vi "Main.vi"   [LabVIEW 2020, in "ClashRoyale.lvclass"]
uses:
  ClashRoyale.lvclass
  support/Popup Loading Toolkit.lvlibp/Handler/Popup Loading Handler.lvclass
types:
  T1 = typedef "InitParameters.ctl" = cluster{"PlayerTag":string}
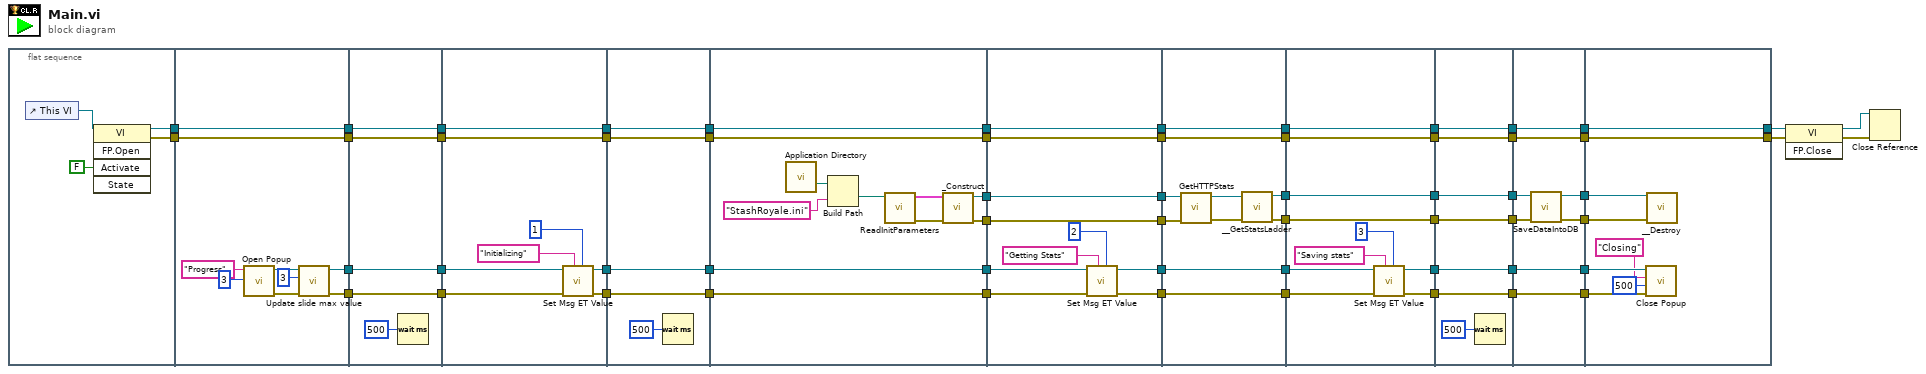
[diagram p0: block diagram]
diagram:
  n1 = flat-sequence {
    tunnel: [w61] -> w16
    tunnel: [w60] -> w5
    tunnel: [w68] -> w38
    tunnel: [w67] -> w36
    tunnel: [w64] -> w17
    tunnel: w16 -> [w64]
    tunnel: [w63] -> w6
    tunnel: w5 -> [w63]
    tunnel: w38 -> [w76]
    tunnel: [w76] -> w37
    tunnel: w36 -> [w75]
    tunnel: [w75] -> w35
    tunnel: [w73] -> w18
    tunnel: w17 -> [w73]
    tunnel: [w72] -> w7
    tunnel: w6 -> [w72]
    tunnel: w37 -> [w84]
    tunnel: w35 -> [w83]
    tunnel: [w80] -> w42
    tunnel: [w79] -> w40
    tunnel: [w78] -> w19
    tunnel: w18 -> [w78]
    tunnel: [w77] -> w8
    tunnel: w7 -> [w77]
    tunnel: w42 -> [w89]
    tunnel: [w89] -> w41
    tunnel: w40 -> [w88]
    tunnel: [w88] -> w39
    tunnel: [w86] -> w20
    tunnel: w19 -> [w86]
    tunnel: [w85] -> w9
    tunnel: w8 -> [w85]
    tunnel: w41 -> [w93]
    tunnel: w39 -> [w92]
    tunnel: [w95] -> w58
    tunnel: [w94] -> w57
    tunnel: [w93] -> w56
    tunnel: [w92] -> w55
    tunnel: [w91] -> w21
    tunnel: w20 -> [w91]
    tunnel: [w90] -> w10
    tunnel: w9 -> [w90]
    tunnel: w58 -> [w110]
    tunnel: w57 -> [w109]
    tunnel: w56 -> [w106]
    tunnel: w55 -> [w105]
    tunnel: [w110] -> w54
    tunnel: [w109] -> w53
    tunnel: [w104] -> w52
    tunnel: [w103] -> w51
    tunnel: [w102] -> w22
    tunnel: w21 -> [w102]
    tunnel: [w101] -> w11
    tunnel: w10 -> [w101]
    tunnel: w54 -> [w116]
    tunnel: w53 -> [w115]
    tunnel: w52 -> [w120]
    tunnel: w51 -> [w119]
    tunnel: [w120] -> w50
    tunnel: [w119] -> w49
    tunnel: [w114] -> w48
    tunnel: [w113] -> w47
    tunnel: [w112] -> w23
    tunnel: w22 -> [w112]
    tunnel: [w111] -> w12
    tunnel: w11 -> [w111]
    tunnel: w50 -> [w126]
    tunnel: w49 -> [w125]
    tunnel: w48 -> [w130]
    tunnel: w47 -> [w129]
    tunnel: [w130] -> w34
    tunnel: [w129] -> w32
    tunnel: [w124] -> w30
    tunnel: [w123] -> w28
    tunnel: [w122] -> w24
    tunnel: w23 -> [w122]
    tunnel: [w121] -> w13
    tunnel: w12 -> [w121]
    tunnel: w34 -> [w137]
    tunnel: [w137] -> w33
    tunnel: w32 -> [w136]
    tunnel: [w136] -> w31
    tunnel: w30 -> [w135]
    tunnel: [w135] -> w29
    tunnel: w28 -> [w134]
    tunnel: [w134] -> w27
    tunnel: [w132] -> w25
    tunnel: w24 -> [w132]
    tunnel: [w131] -> w14
    tunnel: w13 -> [w131]
    tunnel: w33 -> [w143]
    tunnel: w31 -> [w142]
    tunnel: w29 -> [w145]
    tunnel: w27 -> [w144]
    tunnel: [w145] -> w46
    tunnel: [w144] -> w45
    tunnel: [w141] -> w44
    tunnel: [w140] -> w43
    tunnel: [w139] -> w26
    tunnel: w25 -> [w139]
    tunnel: [w138] -> w15
    tunnel: w14 -> [w138]
    tunnel: w46 -> [w151]
    tunnel: w45 -> [w150]
    tunnel: w44 -> [w153]
    tunnel: w43 -> [w152]
    tunnel: w26 -> [w147]
    tunnel: w15 -> [w146]
    tunnel: [w147] -> w2
    tunnel: [w146] -> w1
    frame #0 {
      n2 = control-ref of="This VI"() -> (w59:refnum<vi>)
      n3 = invoke class="VI" method="FP.Open"(reference=w59, "Activate"=FALSE ("Activate?")) -> (reference out=w61:refnum<vi>, error out=w60:errorcluster)  [unwired: 3 in, 3 out]
    }
    frame #1 {
      n4 = call "Open Popup.vi"("Nb Steps"=u32 3, "Title"="Progress") -> ("error out"=w69:errorcluster, "Popup Loading Handler out"=w70:refnum<class "Popup Loading Handler.lvclass">)  [unwired: 8 in]
      n5 = call "Update slide max value.vi"("error in (no error)"=w69, "Slide Max"=u32 3, "Popup Loading Handler in"=w70) -> ("error out"=w67:errorcluster, "Popup Loading Handler out"=w68:refnum<class "Popup Loading Handler.lvclass">)  [unwired: 7 in]
    }
    frame #2 {
      n6 = Wait (ms)(milliseconds to wait=u32 500) -> ()  [unwired: 1 out]
    }
    frame #3 {
      n7 = call "Set Msg ET Value.vi"("New Value"=u32 1, "New Message"="Initializing", "error in (no error)"=w83, "Popup Loading Handler in"=w84) -> ("error out"=w79:errorcluster, "Popup Loading Handler out"=w80:refnum<class "Popup Loading Handler.lvclass">)  [unwired: 6 in]
    }
    frame #4 {
      n8 = Wait (ms)(milliseconds to wait=u32 500) -> ()  [unwired: 1 out]
    }
    frame #5 {
      n9 = call <vilib>:"Application Directory.vi"() -> ("Application Directory"=w99:path)
      n10 = Build Path(base path=w99, name or relative path="StashRoyale.ini" ("Title")) -> (appended path=w98:path)
      n11 = call "ReadInitParameters.vi"("INI Filepath"=w98) -> ("error out"=w100:errorcluster, "Init Parameters"=w97:T1)  [unwired: 9 in]
      n12 = call "_Construct.vi"("error in (no error)"=w100, "Init Parameters"=w97) -> ("error out"=w95:errorcluster, "ClashRoyale out"=w94:refnum<class "ClashRoyale.lvclass">)  [unwired: 8 in]
    }
    frame #6 {
      n13 = call "Set Msg ET Value.vi"("New Value"=u32 2, "New Message"="Getting Stats", "error in (no error)"=w105, "Popup Loading Handler in"=w106) -> ("error out"=w103:errorcluster, "Popup Loading Handler out"=w104:refnum<class "Popup Loading Handler.lvclass">)  [unwired: 6 in]
    }
    frame #7 {
      n14 = call "GetHTTPStats.vi"("error in (no error)"=w116, "ClashRoyale in"=w115) -> ("error out"=w118:errorcluster, "ClashRoyale out"=w117:refnum<class "ClashRoyale.lvclass">)  [unwired: 8 in]
      n15 = call "__GetStatsLadder.vi"("error in (no error)"=w118, "ClashRoyale in"=w117) -> ("error out"=w114:errorcluster, "ClashRoyale out"=w113:refnum<class "ClashRoyale.lvclass">)  [unwired: 8 in]
    }
    frame #8 {
      n16 = call "Set Msg ET Value.vi"("New Value"=u32 3, "New Message"="Saving stats", "error in (no error)"=w125, "Popup Loading Handler in"=w126) -> ("error out"=w123:errorcluster, "Popup Loading Handler out"=w124:refnum<class "Popup Loading Handler.lvclass">)  [unwired: 6 in]
    }
    frame #9 {
      n17 = Wait (ms)(milliseconds to wait=u32 500) -> ()  [unwired: 1 out]
    }
    frame #10 {
      n18 = call "SaveDataIntoDB.vi"("error in (no error)"=w143, "ClashRoyale in"=w142) -> ("error out"=w141:errorcluster, "ClashRoyale out"=w140:refnum<class "ClashRoyale.lvclass">)  [unwired: 8 in]
    }
    frame #11 {
      n19 = call "Close Popup.vi"("error in (no error)"=w150, "Wait (200 ms)"=u32 500, "Last Message"="Closing", "Popup Loading Handler in"=w151) -> ()  [unwired: 7 in, 1 out]
      n20 = call "__Destroy.vi"("error in (no error)"=w153, "ClashRoyale in"=w152) -> ()  [unwired: 9 in, 1 out]
    }
  }
  n21 = invoke class="VI" method="FP.Close"(reference=w2, error in=w1) -> (reference out=w4:refnum<vi>, error out=w3:errorcluster)  [unwired: 1 in, 1 out]
  n22 = Close Reference(reference=w4, error in (no error)=w3) -> ()  [unwired: 1 out]
